vi "Stream Reader.vi"(7 "Popup? (F)":bool, 8 "error in (no error)":errorcluster, 10 "Signals in":refnum<class "ISignal.lvclass">[](array[class])) -> (0 "error out":errorcluster)   [LabVIEW 2022 SP3, in "StreamReader.lvlib"]
uses:
  <instrlib>/openDAQ/Examples/StreamReader/StreamReader.lvlib
  <instrlib>/openDAQ/Public/TypeDef/DomainMetadata.ctl
  <instrlib>/openDAQ/Public/Classes/ISignal/ISignal.lvclass
  C:/Program Files (x86)/National Instruments/LabVIEW 2022/instr.lib/openDAQ/Public/Classes/IComponent/IComponent.lvclass
  C:/Program Files (x86)/National Instruments/LabVIEW 2022/instr.lib/openDAQ/Public/Classes/IBaseObject/IBaseObject.lvclass
  <instrlib>/openDAQ/Examples/StreamReader/TypeDef/State.ctl
  <instrlib>/openDAQ/Public/Classes/IInstance/IInstance.lvclass
  C:/Program Files (x86)/National Instruments/LabVIEW 2022/instr.lib/openDAQ/Public/Classes/IDevice/IDevice.lvclass
  <instrlib>/openDAQ/Public/Classes/IDevice/IDevice.lvclass
  <instrlib>/openDAQ/Public/Classes/IStreamReader/IStreamReader.lvclass
  C:/Program Files (x86)/National Instruments/LabVIEW 2022/instr.lib/openDAQ/Public/Classes/IReader/IReader.lvclass
  <instrlib>/openDAQ/Public/Classes/IBaseObject/Polymorphic/queryInterface/queryDataDescriptorInterface.vi
  <instrlib>/openDAQ/Public/Classes/daqCoreTypes/IDict/IDict.lvclass
  <instrlib>/openDAQ/Public/Classes/IBaseObject/IBaseObject.lvclass
  <instrlib>/openDAQ/Public/Classes/IDataDescriptor/IDataDescriptor.lvclass
  <instrlib>/openDAQ/Public/Classes/IEventPacket/IEventPacket.lvclass
  <instrlib>/openDAQ/Public/Classes/daqUtils/daqUtils.lvlib
  <instrlib>/openDAQ/openDAQ.lvlib
  <instrlib>/openDAQ/Public/Classes/IReaderStatus/IReaderStatus.lvclass
  <instrlib>/openDAQ/Public/Classes/IComponent/IComponent.lvclass
  <instrlib>/openDAQ/Public/Classes/IReader/IReader.lvclass
panel:
  in  "Btn:StopMeasurement":bool
  in  "Online Buffer":i32=1000
  in  "Btn:StartMeasurement":bool
  in  "Btn:Stop":bool
  out "Iteration":i32
  out "DomainMetadata":T1
  in  "Global ID's":i32(listbox)
  out "XY Graph":T2(graph)
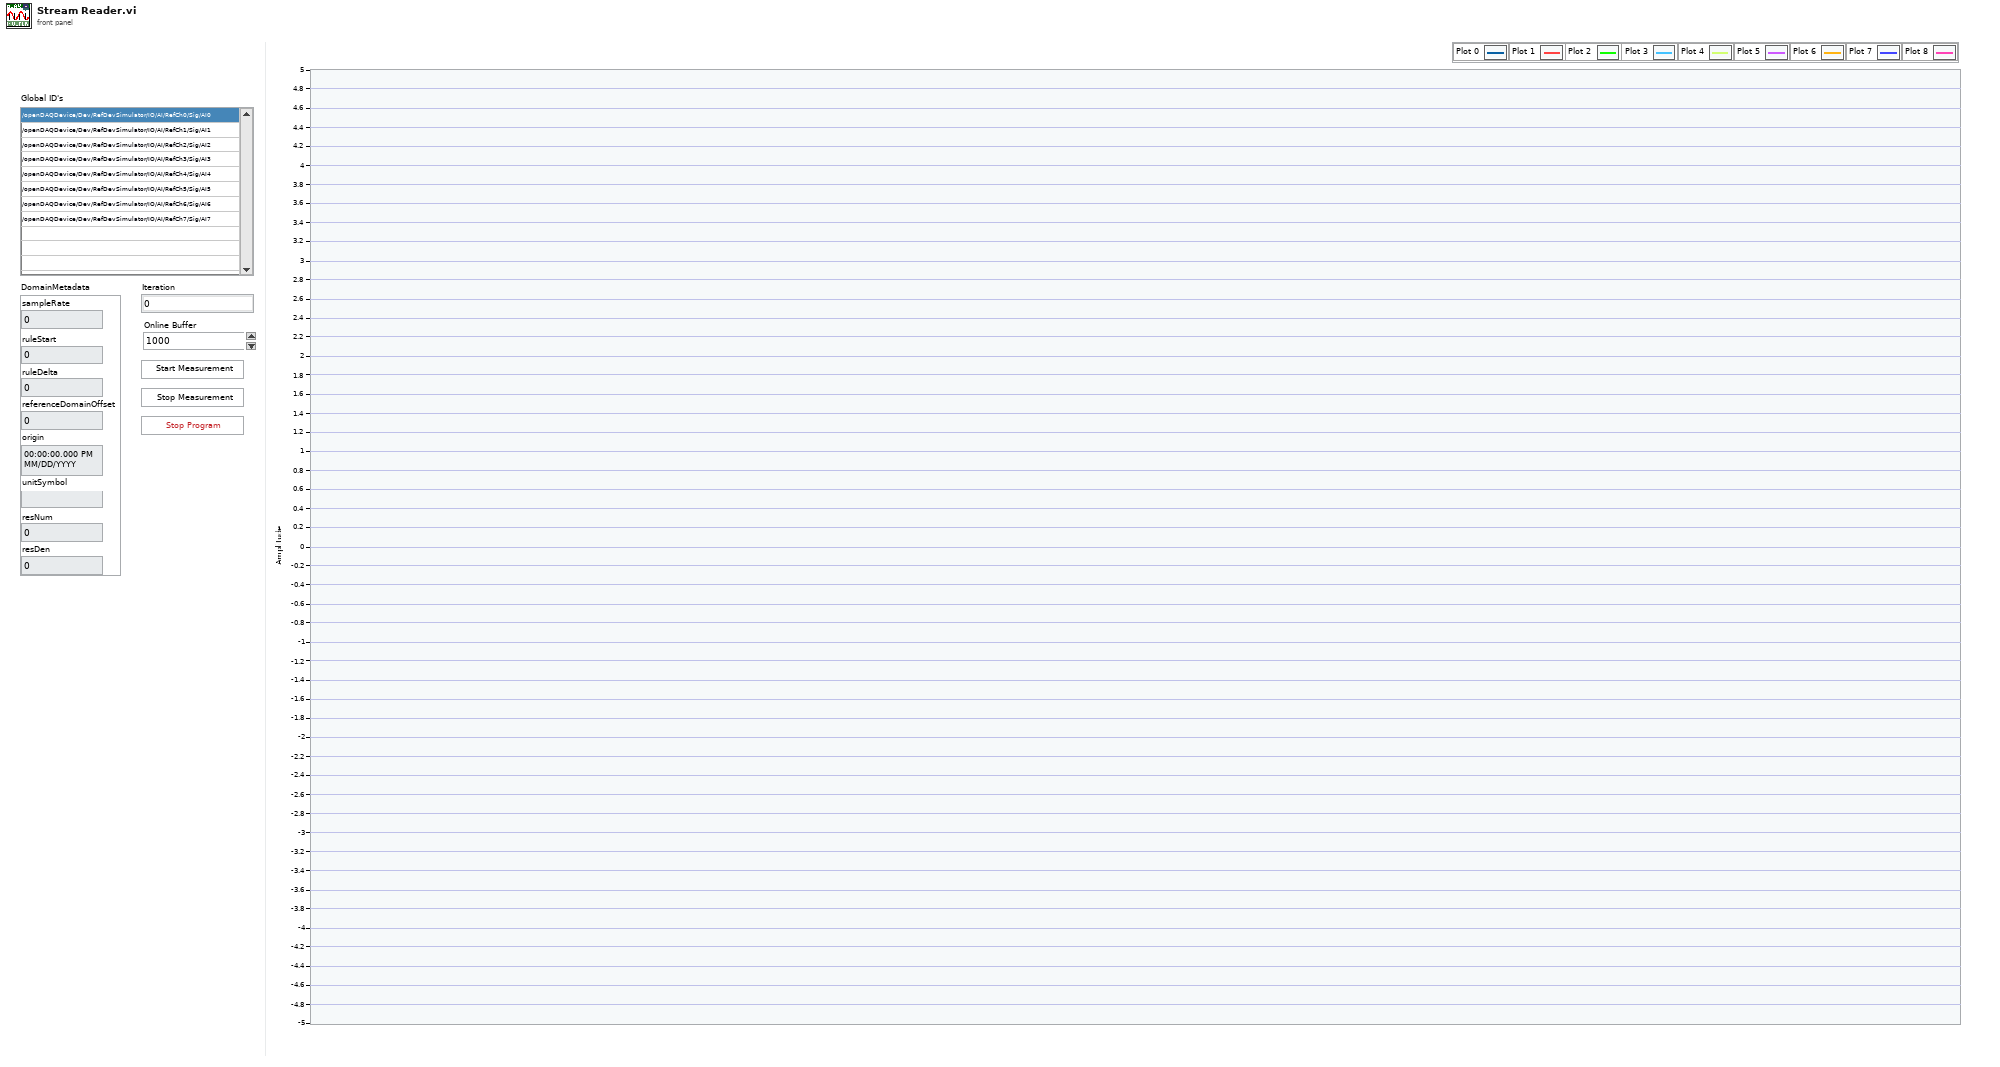
[diagram p1: front panel]
types:
  T1 = typedef "openDAQ.lvlib/DomainMetadata.ctl" = cluster{"sampleRate":i64, "ruleStart":i64, "ruleDelta":i64, "referenceDomainOffset":i64, "origin":timestamp, "unitSymbol":string, "resNum":i64, "resDen":i64}
  T2 = cluster{"Waveform Graph":timestamp[], "Waveform Graph":dbl[]}
  T3 = cluster{"Simulator":refnum<class "IInstance.lvclass">, "Instance":refnum<class "IInstance.lvclass">, "ConnectedDevice":refnum<class "IDevice.lvclass">, "Signals":refnum<class "ISignal.lvclass">[], "ChannelCount":i32, "StreamReader":refnum<class "IStreamReader.lvclass">}
  T4 = typedef "StreamReader.lvlib/State.ctl" = enum16{"INIT", "- SIMULATOR.setup", "IDLE", "- DAQ.start", "- DAQ.read", "- DAQ.end", "STOP", "ERROR"}
  T5 = enum16{"init", "read", "set sampleRate", "set ruleStart", "set ruleDelta", "set referenceDomainOffset", "set origin", "set unitSymbol", "set resNum", "set resDen", " calculate sampleRate"}
  T6 = enum8{"Enabled", "Disabled", "Disabled and Grayed Out"}
  T7 = cluster{"Value Buffer":dbl[], "Domain Buffer":i64[]}
  T8 = typedef "openDAQ.lvlib/ReadStatus.ctl" = u16
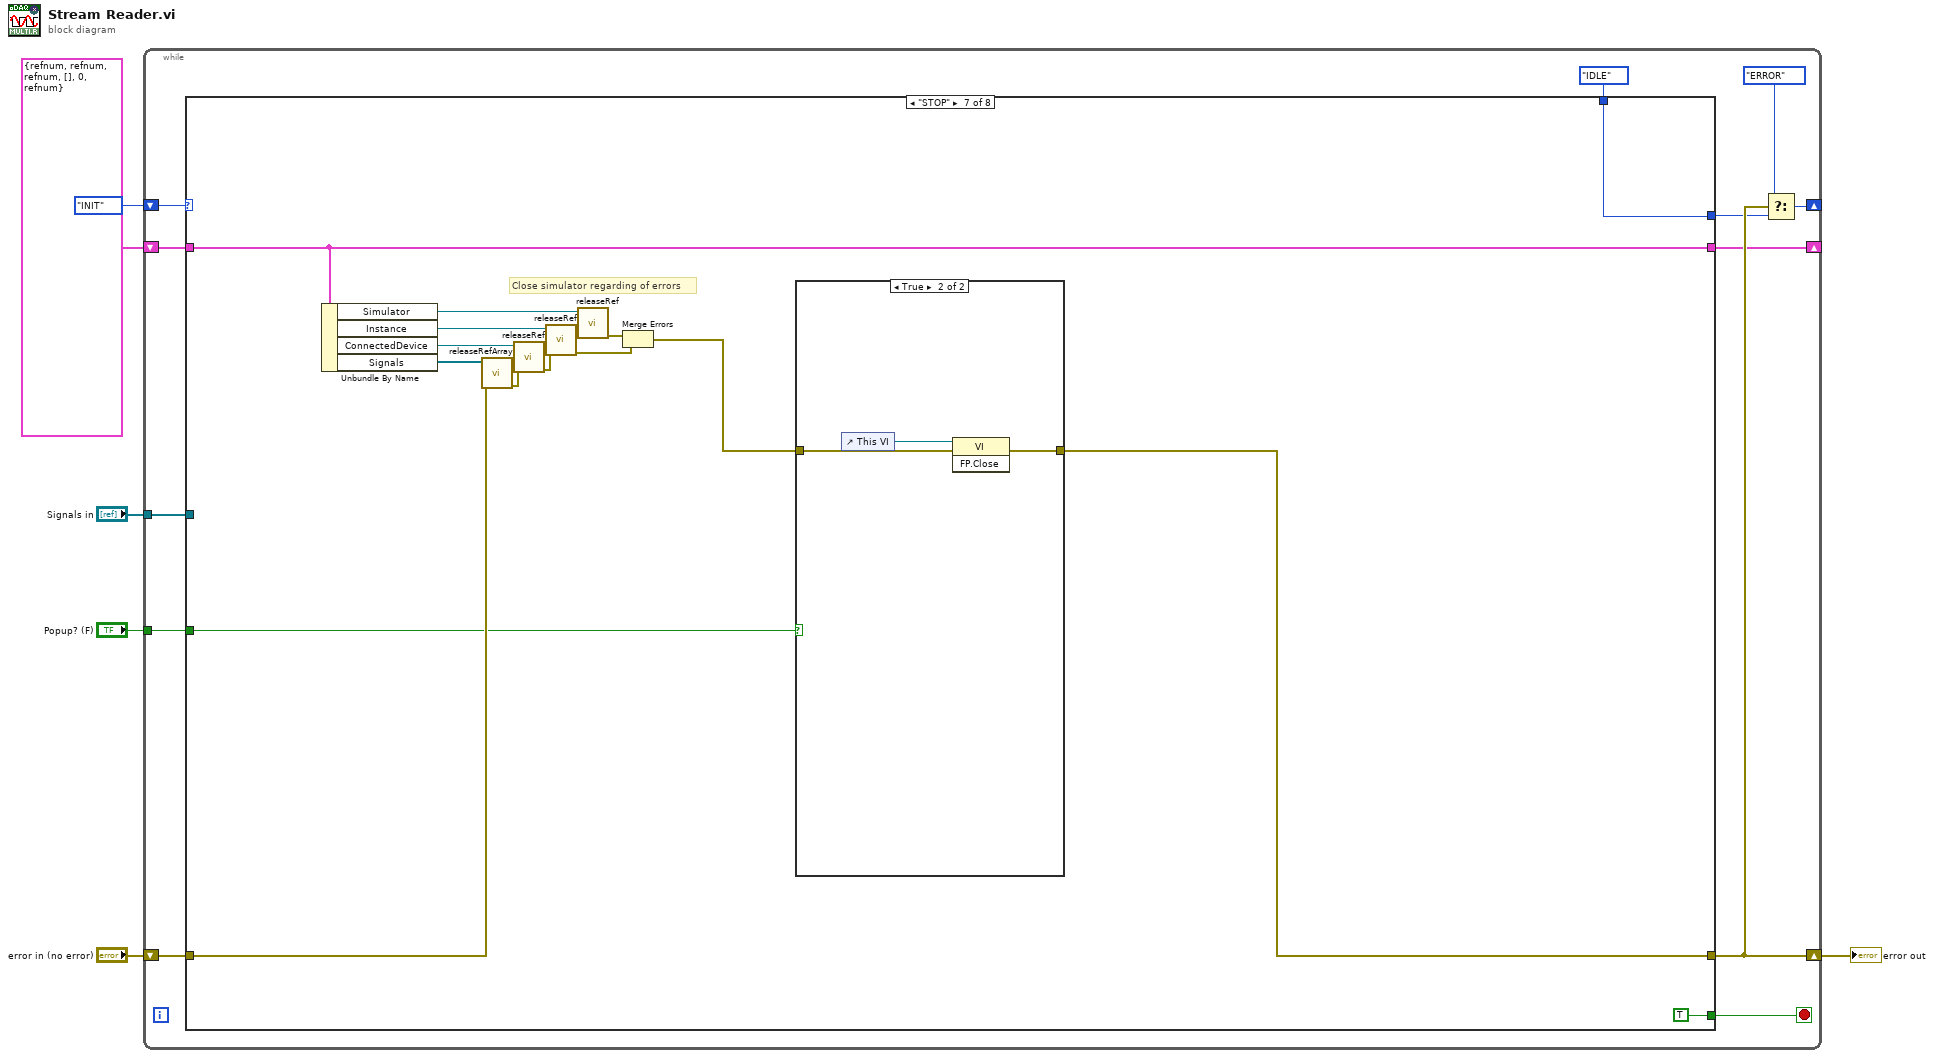
[diagram p0: block diagram]
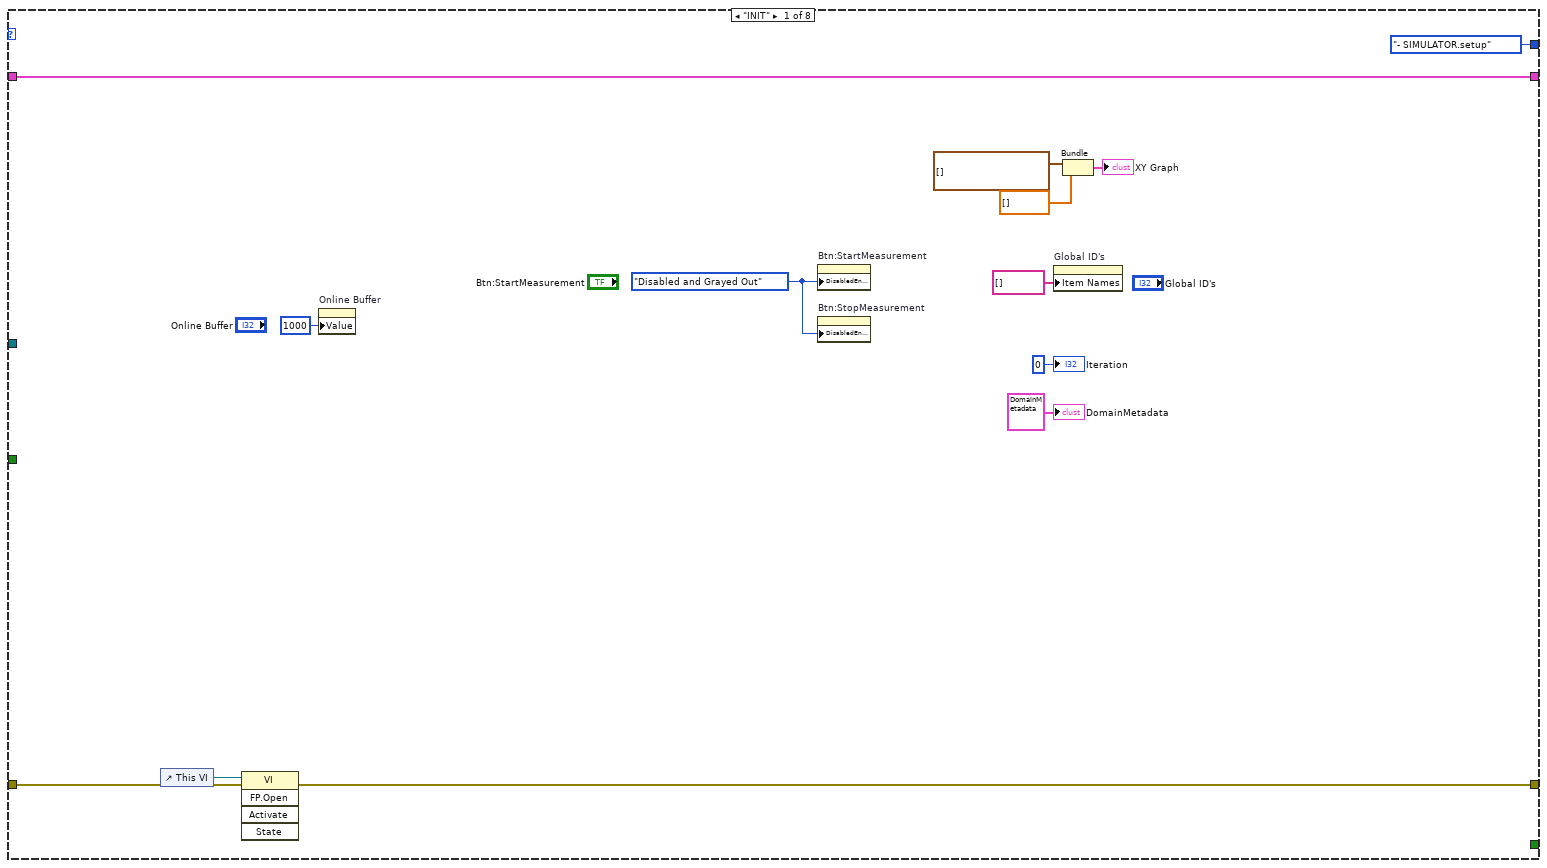
[diagram p2: hidden frame]
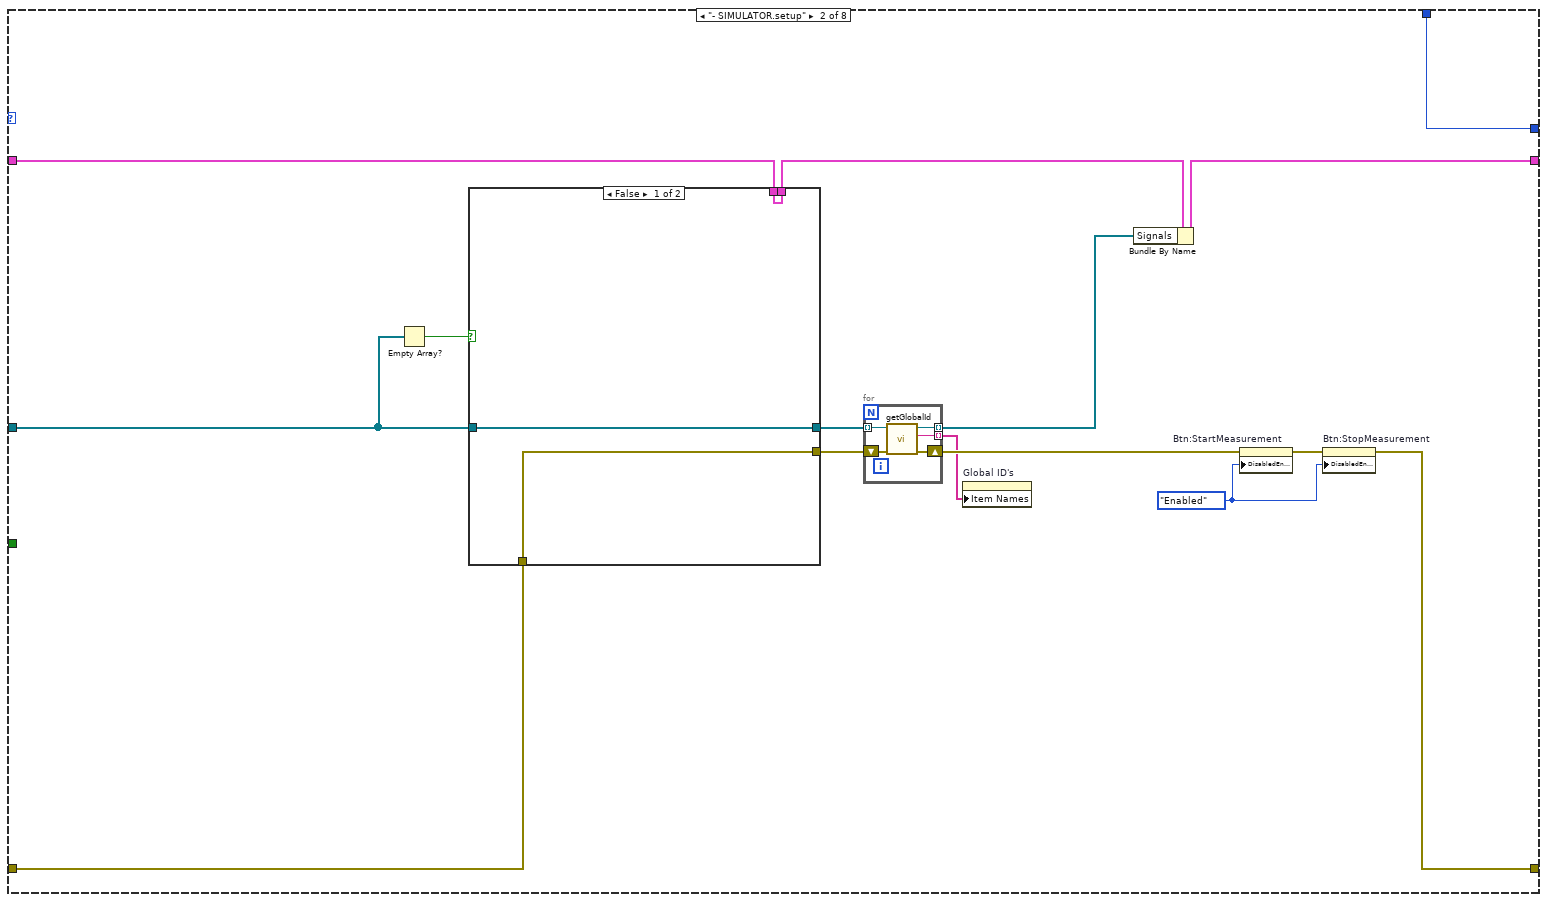
[diagram p3: hidden frame]
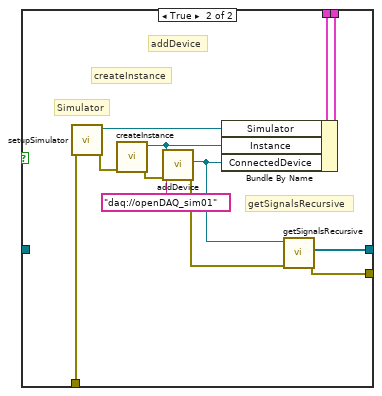
[diagram p4: hidden frame]
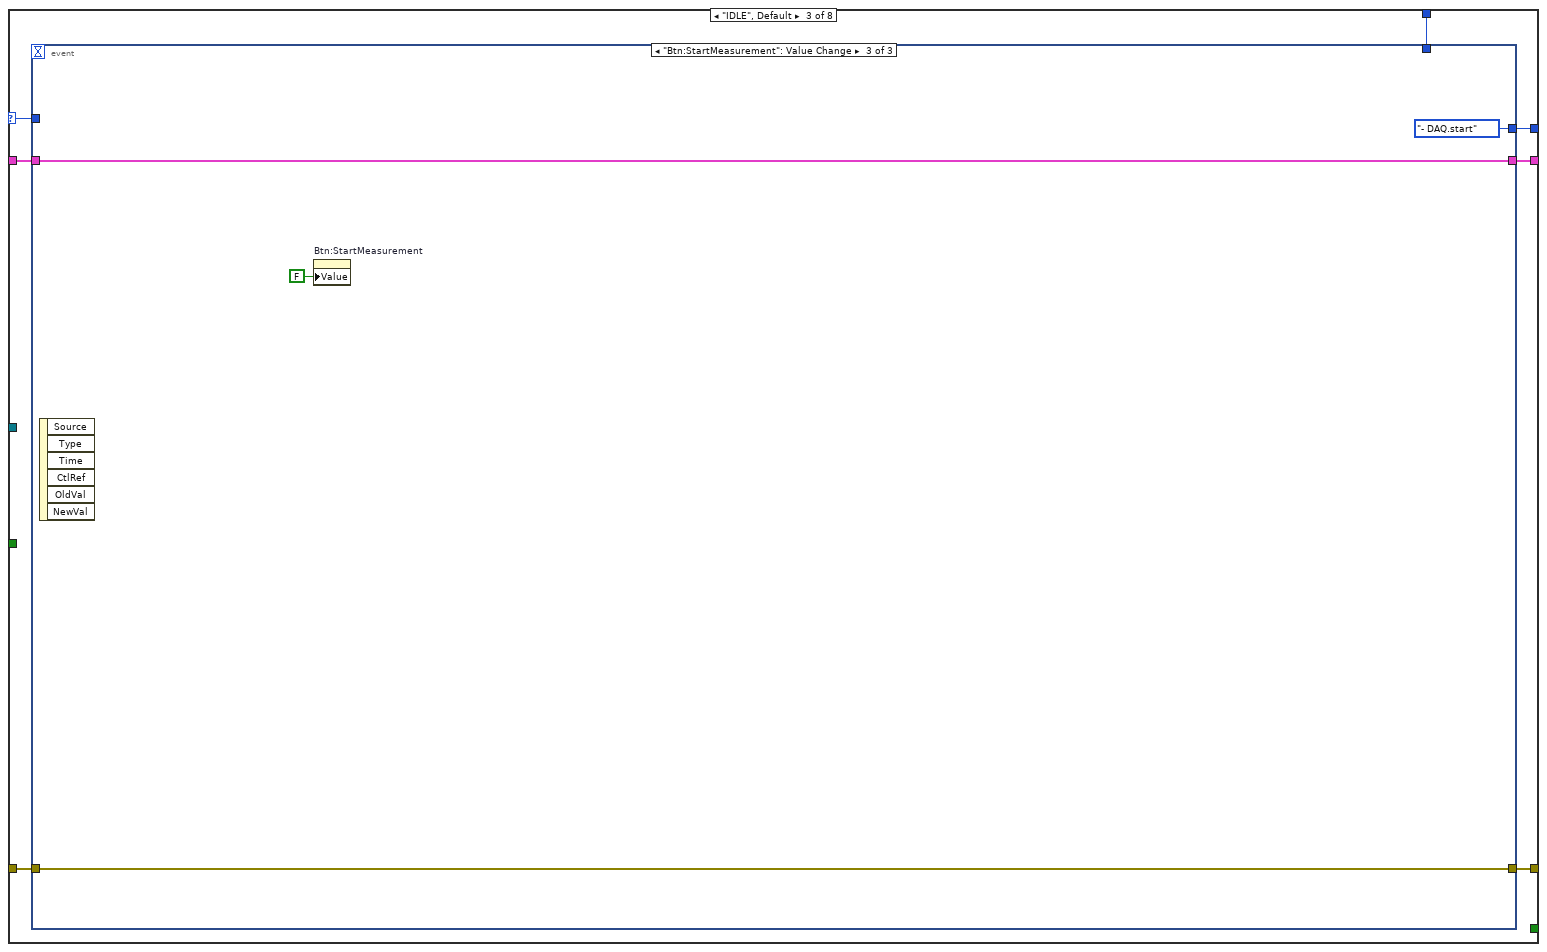
[diagram p5: hidden frame]
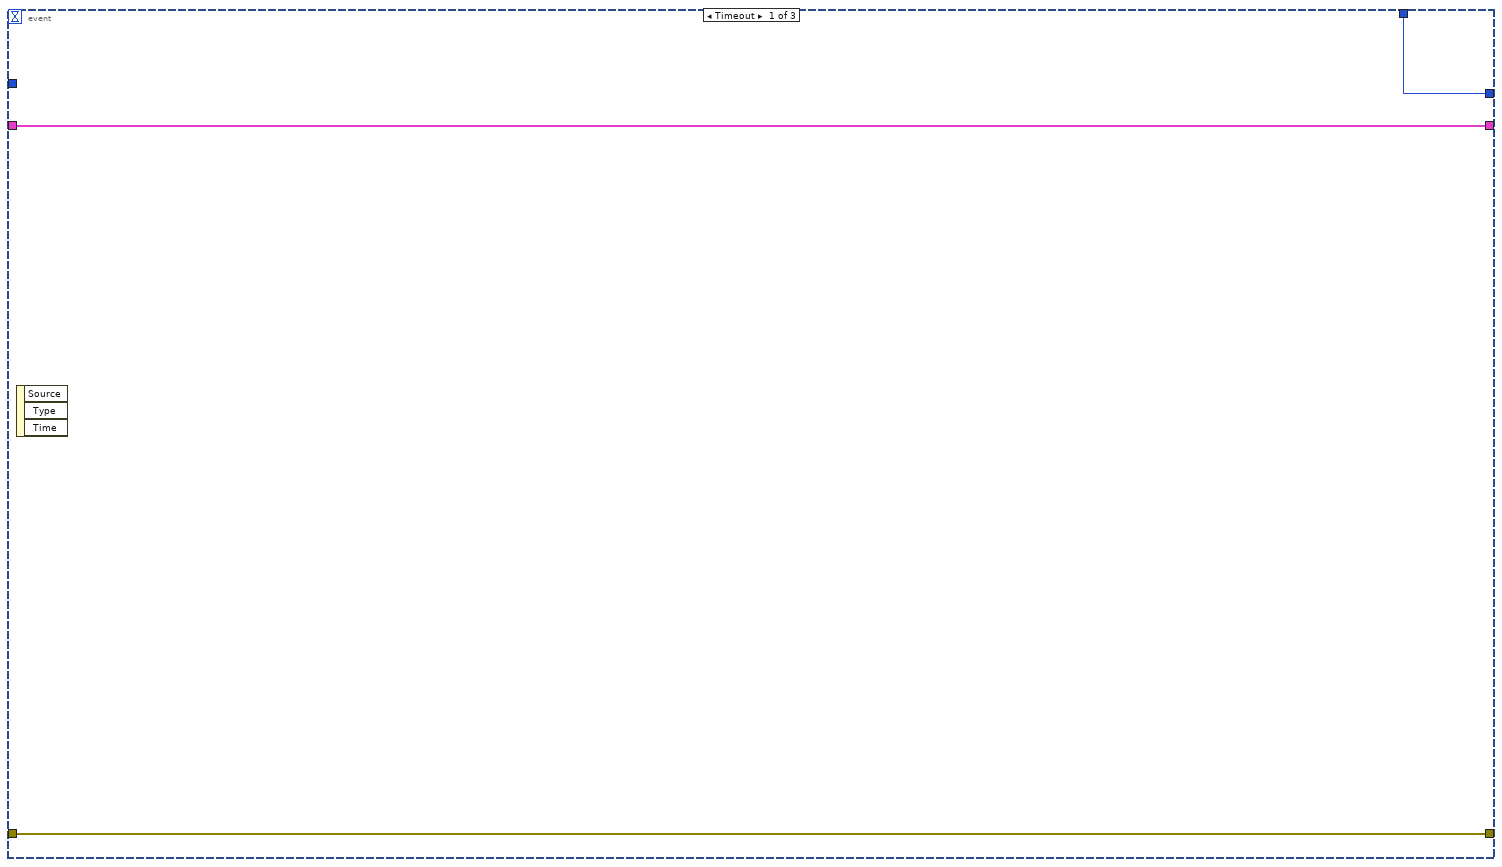
[diagram p6: hidden frame]
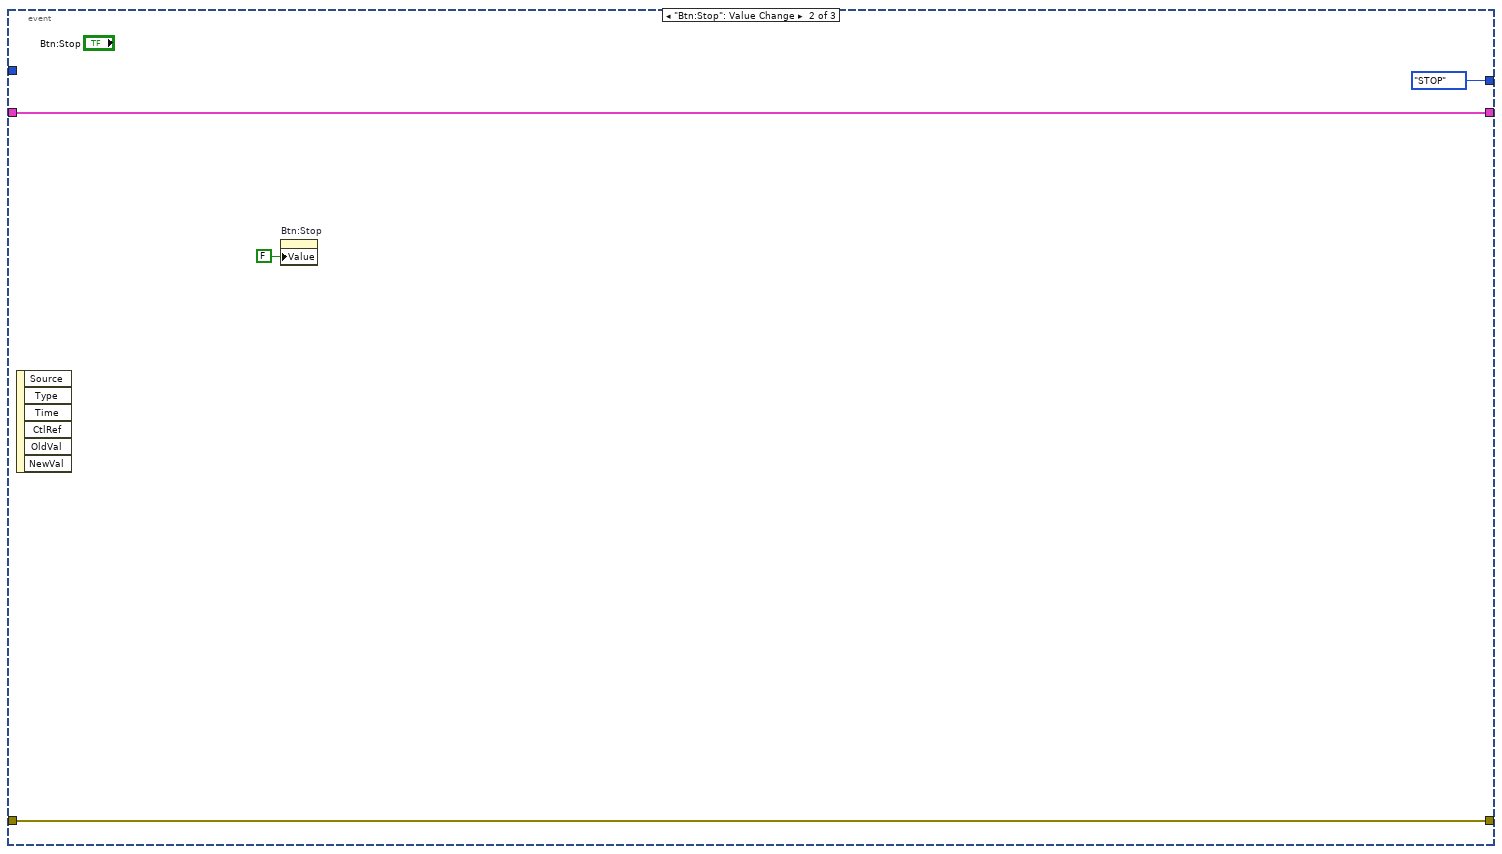
[diagram p7: hidden frame]
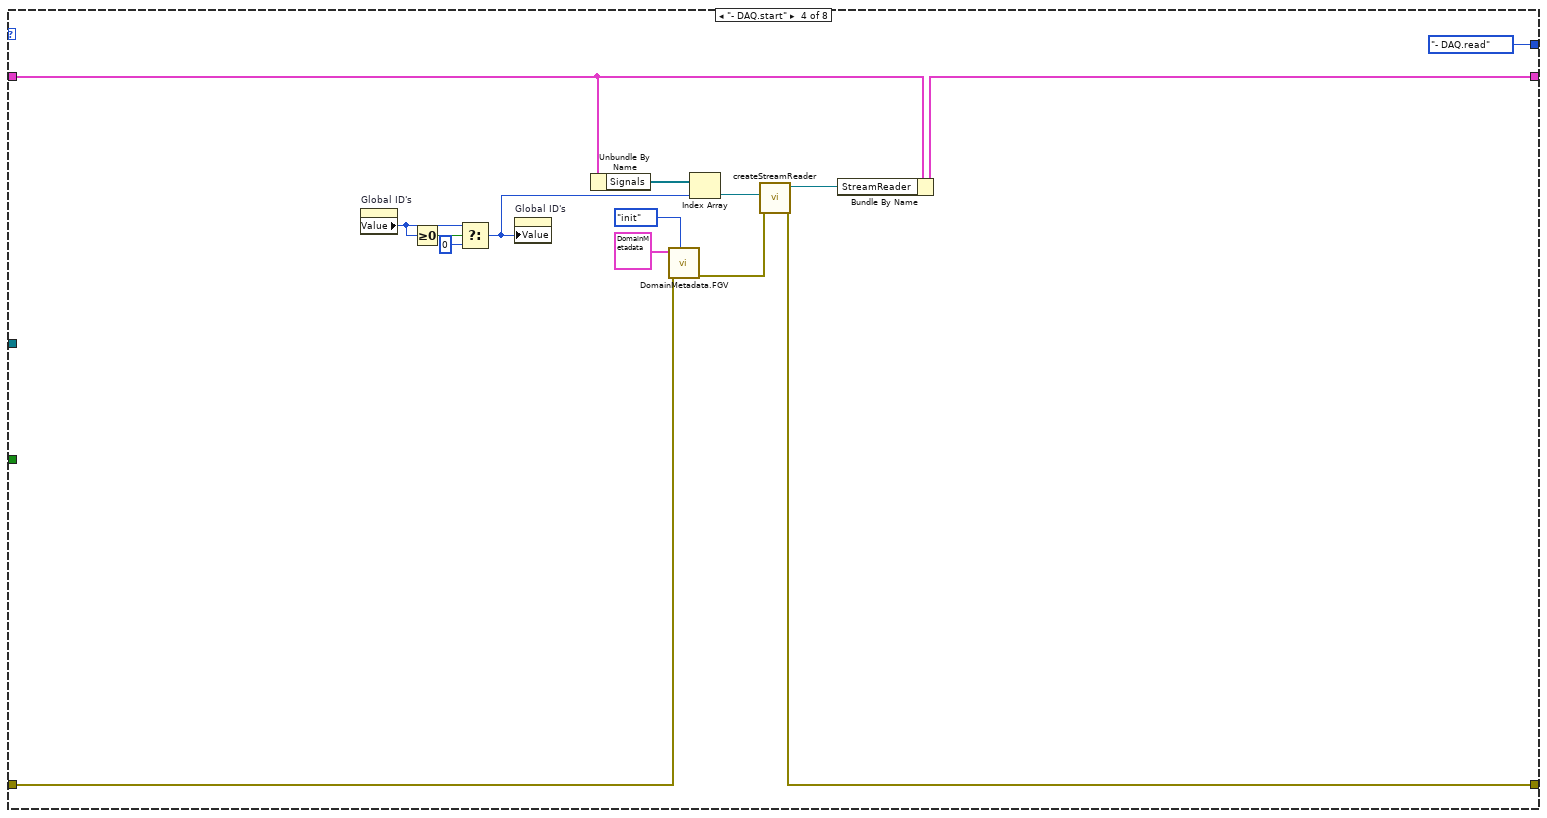
[diagram p8: hidden frame]
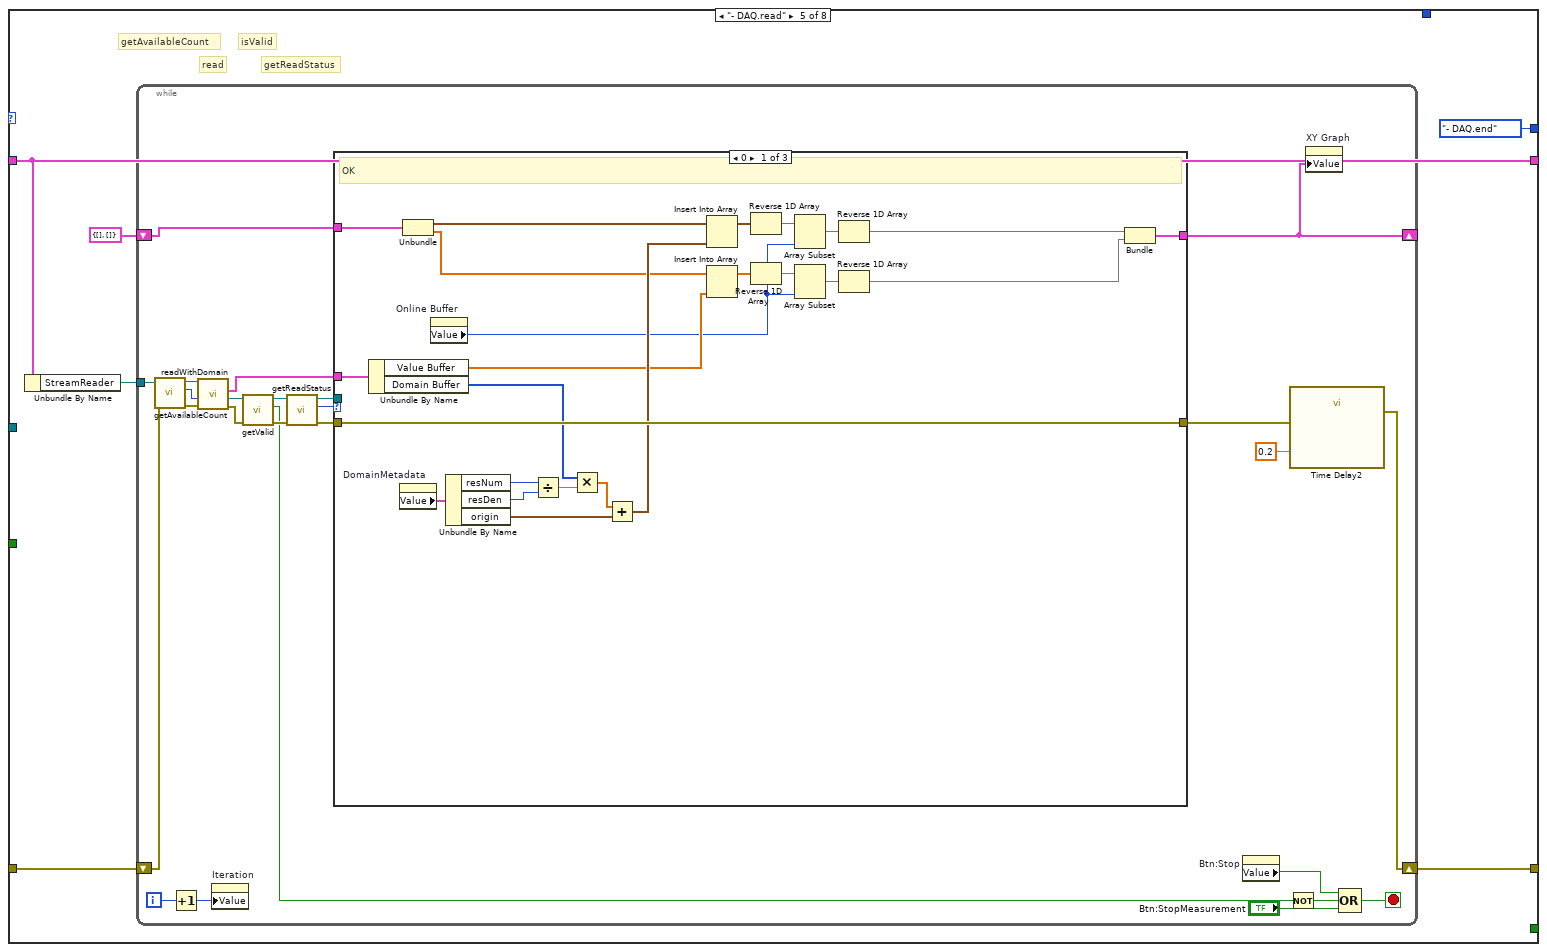
[diagram p9: hidden frame]
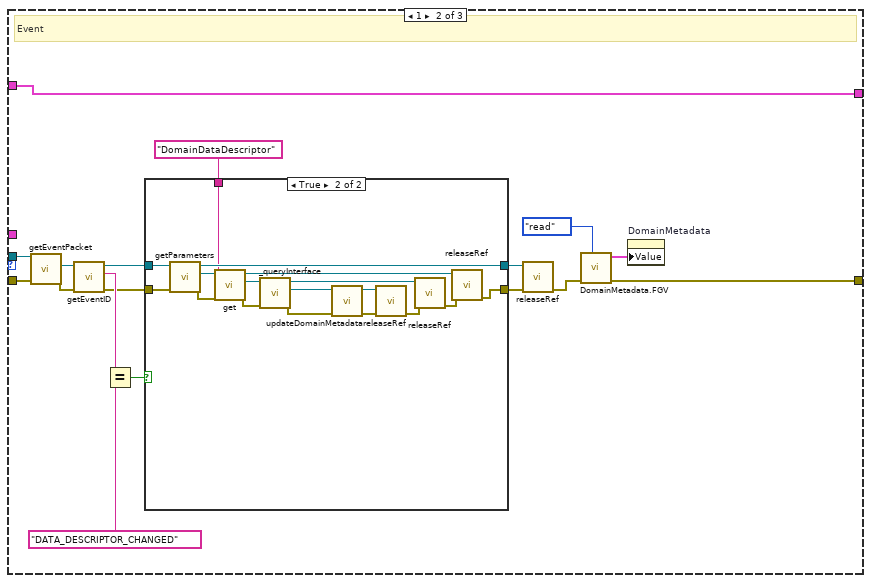
[diagram p10: hidden frame]
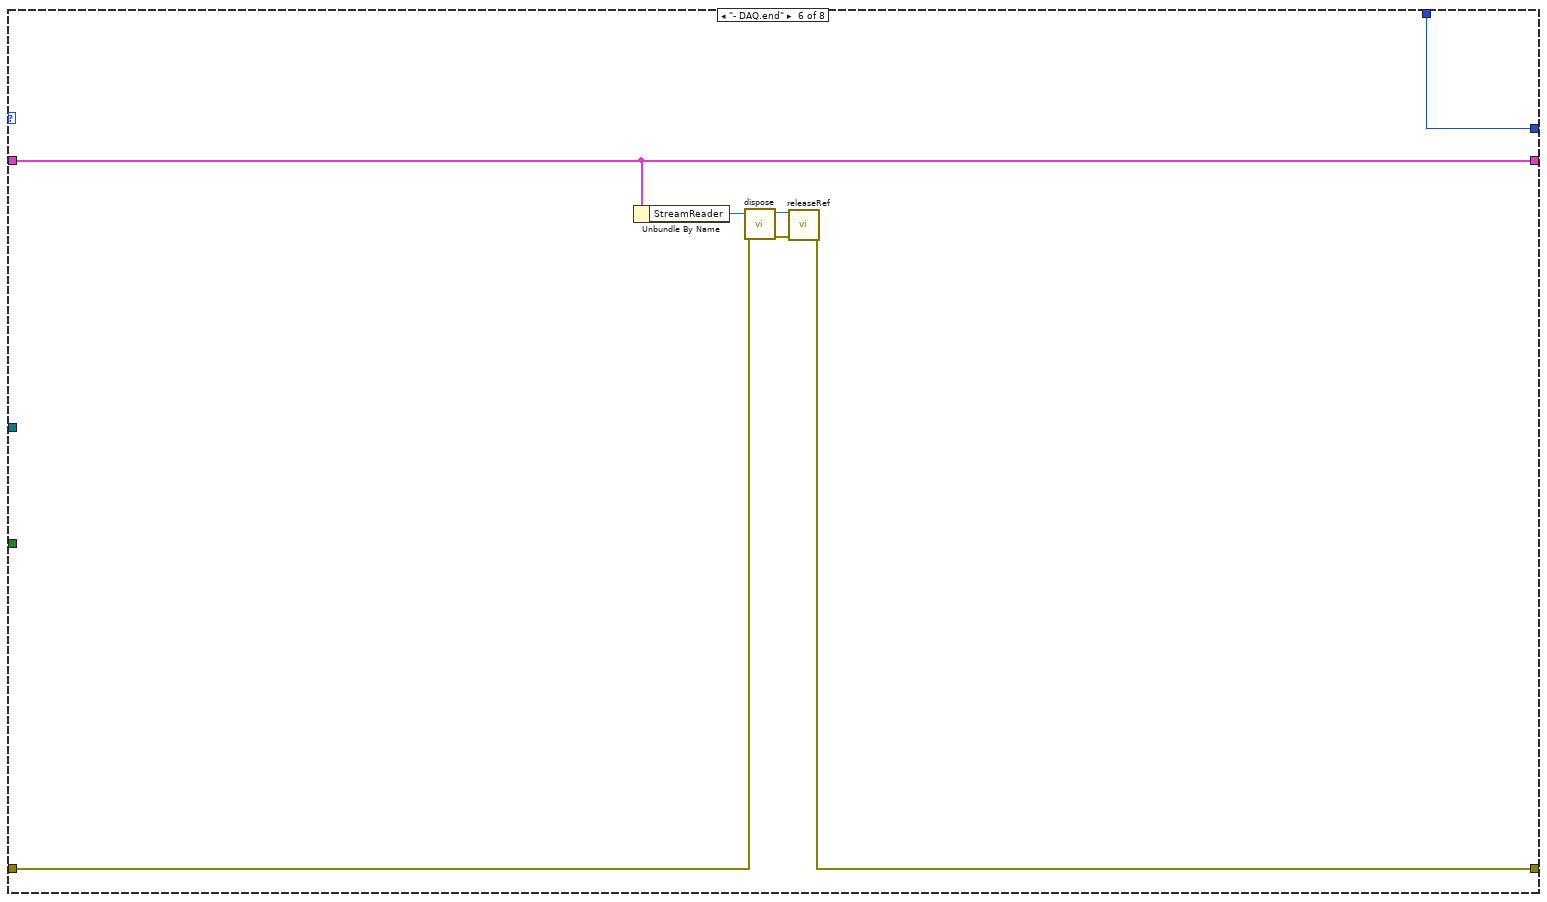
[diagram p13: hidden frame]
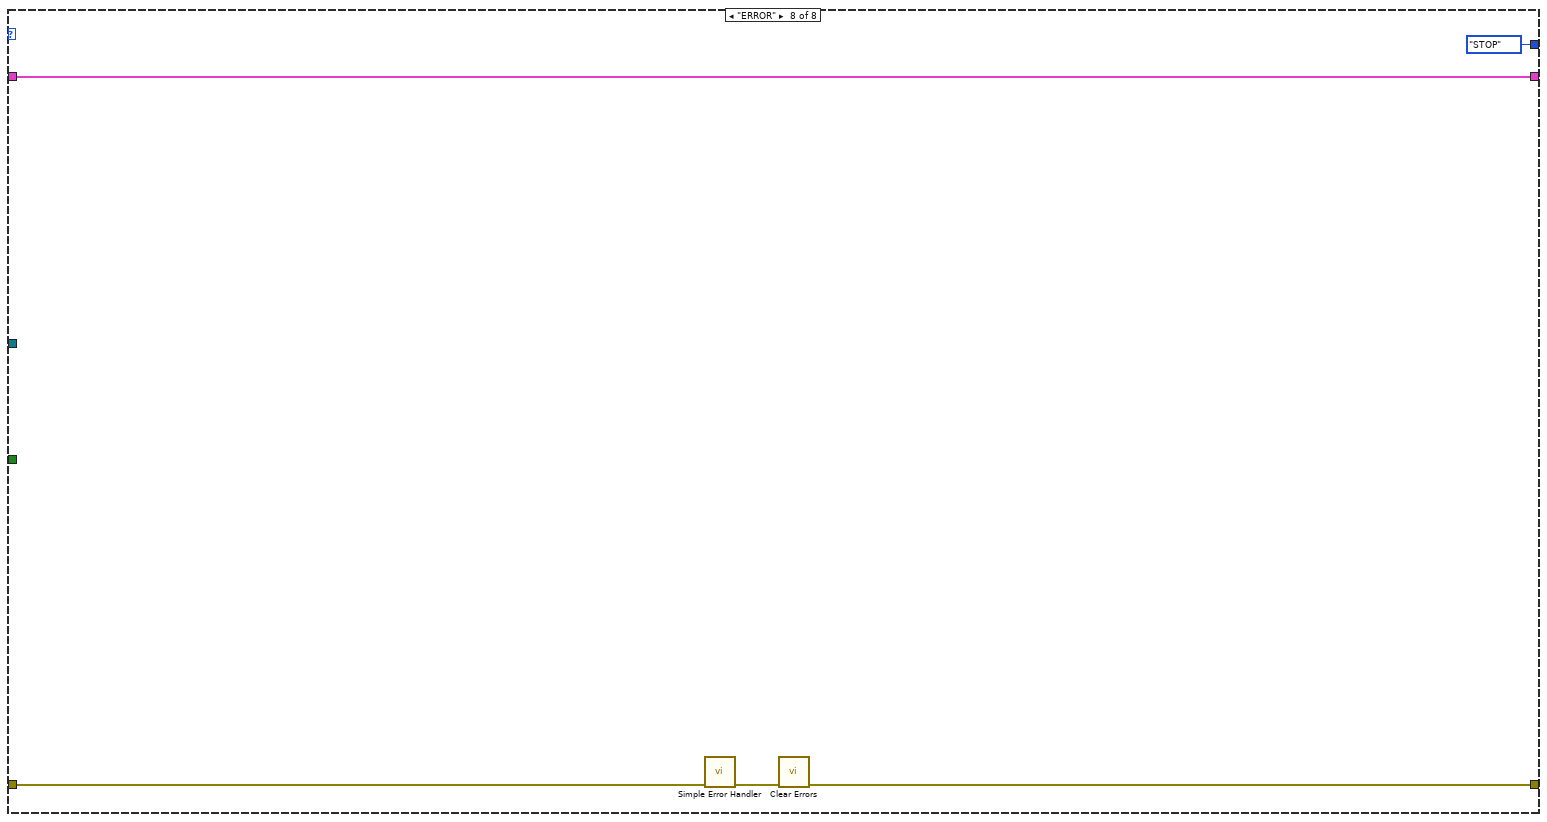
[diagram p15: hidden frame]
diagram:
  n1 = while {
    shift-right: [w11] -> _
    shift-left: State."INIT" -> [w17]
    shift-right: [w18] -> w2
    shift-left: "error in (no error)" -> [w14]
    shift-right: [w12] -> _
    shift-left: T3 {"Simulator"=refnum, "Instance"=refnum, "ConnectedDevice"=refnum, "Signals"=[], "ChannelCount"=0, "StreamReader"=refnum} -> [w13]
    tunnel: "Signals in" -> [w8]
    tunnel: "Popup? (F)" -> [w7]
    stop <- w16 stop-if-true
    n2 = case shown="\"STOP\"" w17 {
      selector: w17 -> [_ _ w73 _ _ _ _ _]
      tunnel: [State."- SIMULATOR.setup" w44 w71 State."- DAQ.read" State."- DAQ.end" w199 w203 State."STOP"] -> w10
      tunnel: [_ _ _ _ _ _ TRUE _] -> w16
      tunnel: State."IDLE" -> [_ w44 w72 _ _ w199 w203 _]
      tunnel: w14 -> [w24 w45 w70 w86 w103 w195 w205 w221]
      tunnel: [w23 w39 w69 w98 w102 w197 w200 w220] -> w18
      tunnel: w13 -> [w31 w43 w68 w95 w104 w198 w213 w223]
      tunnel: [w31 w41 w67 w93 w104 w198 w213 w223] -> w12
      tunnel: w8 -> [_ w36 _ _ _ _ _ _]
      tunnel: w7 -> [_ _ _ _ _ _ w202 _]
      frame "INIT" {
        w26 = T6."Disabled and Grayed Out" ("Disabled")
        n3 = control-ref of="This VI"() -> (w25:refnum<vi>)
        n4 = invoke class="VI" method="FP.Open"(reference=w25, error in=w24) -> (error out=w23:errorcluster)  [unwired: 3 in, 4 out]
        n5 = property on="Online Buffer" class="DigNum (strict)"("Value"=1000 ("Online Buffer")) -> ()  [unwired: 2 in, 2 out]
        n6 = property on="Btn:StartMeasurement" class="Bool (strict)"("DisabledEnum"=w26) -> ()  [unwired: 2 in, 2 out]
        n7 = property on="Btn:StopMeasurement" class="Bool"("DisabledEnum"=w26) -> ()  [unwired: 2 in, 2 out]
        n8 = property on="Global ID's" class="LstBox (strict)"("Item Names"=string[] [] ("Global ID's")) -> ()  [unwired: 2 in, 2 out]
        n9 = Bundle("Waveform Graph"=timestamp[] [], "Waveform Graph"=dbl[] []) -> (→"XY Graph":T2)  [unwired: 1 in]
        "Iteration" <- 0 ("Iteration")
        "DomainMetadata" <- T1 {"sampleRate"=0, "ruleStart"=0, "ruleDelta"=0, "referenceDomainOffset"=0, "origin"=timestamp(0 s since 1904-01-01), "unitSymbol"="", "resNum"=0, "resDen"=0} ("DomainMetadata")
      }
      frame "- SIMULATOR.setup" {
        w38 = T6."Enabled" ("Disabled")
        n10 = Empty Array?(array=w36) -> (empty?=w37:bool)
        n11 = case shown="False" w37 {
          tunnel: w45 -> [w53 w66]
          tunnel: w43 -> [w54 w60]
          tunnel: [w52 w56] -> w34
          tunnel: [w54 w57] -> w42
          tunnel: [w53 w55] -> w33
          tunnel: w36 -> [w52 _]
          frame False {
          }
          frame True {
            # "Simulator"
            # "addDevice"
            # "createInstance"
            # "getSignalsRecursive"
            n12 = call <instrlib>:"setupSimulator.vi"("error in (no error)"=w66) -> ("error out"=w63:errorcluster, "IInstance out"=w62:refnum<class "IInstance.lvclass">)  [unwired: 9 in]
            n13 = call <instrlib>:"createInstance.vi"("error in (no error)"=w63) -> ("error out"=w65:errorcluster, "IInstance out"=w61:refnum<class "IInstance.lvclass">)  [unwired: 9 in]
            n14 = call <instrlib>:"addDevice.vi"("error in (no error)"=w65, "ConnectionString in"="daq://openDAQ_sim01" ("modulePath"), "IDevice in"=w61) -> ("error out"=w59:errorcluster, "ConnectedDevice out"=w58:refnum<class "IDevice.lvclass">)  [unwired: 6 in, 1 out]
            n15 = Bundle By Name(cluster=w60, "Simulator"=w62, "Instance"=w61, "ConnectedDevice"=w58) -> (w57:T3)
            n16 = call <instrlib>:"getSignalsRecursive.vi"("error in (no error)"=w59, "IDevice in"=w58) -> ("error out"=w55:errorcluster, "Available Sigals out"=w56:refnum<class "ISignal.lvclass">[])  [unwired: 7 in, 1 out]
          }
        }
        n17 = for {
          tunnel: w34 -> [w51] mode=indexing
          tunnel: [w50] -> w32 mode=indexing
          tunnel: [w47] -> w35 mode=indexing
          shift-right: [w48] -> w46
          shift-left: w33 -> [w49]
          n18 = call <instrlib>:"getGlobalId.vi"("error in (no error)"=w49, "IComponent in"=w51) -> ("error out"=w48:errorcluster, "GlobalId out"=w47:string, "IComponent out"=w50:refnum<class "ISignal.lvclass">)  [unwired: 7 in]
        }
        n19 = property on="Global ID's" class="LstBox (strict)"("Item Names"=w35) -> ()  [unwired: 2 in, 2 out]
        n20 = Bundle By Name(cluster=w42, "Signals"=w32) -> (w41:T3)
        n21 = property on="Btn:StartMeasurement" class="Bool (strict)"(error in=w46, "DisabledEnum"=w38) -> (error out=w40:errorcluster)  [unwired: 1 in, 1 out]
        n22 = property on="Btn:StopMeasurement" class="Bool"(error in=w40, "DisabledEnum"=w38) -> (error out=w39:errorcluster)  [unwired: 1 in, 1 out]
      }
      frame "IDLE", Default {
        n23 = event shown="[2] \"Btn:StartMeasurement\": Value Change" {
          selector: _ -> [_ _ _]
          dyn-events: _ -> [_ _ _]
          timeout: _ -> [_ _ _]
          tunnel: w73 -> [_ _ _]
          tunnel: [w76 State."STOP" State."- DAQ.start"] -> w71
          tunnel: w72 -> [w76 _ _]
          tunnel: w70 -> [w75 w80 w82]
          tunnel: [w75 w80 w82] -> w69
          tunnel: w68 -> [w74 w79 w83]
          tunnel: [w74 w79 w83] -> w67
          event Timeout {
            n24 = event-data() -> ()  [unwired: 1 in, 3 out]
          }
          event "Btn:Stop": Value Change {
            n25 = event-data() -> ()  [unwired: 1 in, 6 out]
            n26 = property on="Btn:Stop" class="Bool (strict)"("Value"=FALSE ("Btn:Stop")) -> ()  [unwired: 2 in, 2 out]
          }
          event "Btn:StartMeasurement": Value Change {
            n27 = event-data() -> ()  [unwired: 1 in, 6 out]
            n28 = property on="Btn:StartMeasurement" class="Bool (strict)"("Value"=FALSE ("Btn:StartMeasurement")) -> ()  [unwired: 2 in, 2 out]
          }
        }
      }
      frame "- DAQ.start" {
        n29 = property on="Global ID's" class="LstBox (strict)"() -> ("Value"=w91:i32)  [unwired: 2 in, 2 out]
        n30 = Greater Or Equal To 0?(x=w91) -> (x >= 0?=w92:bool)
        n31 = Select(t=w91, s=w92, f=0) -> (s? t:f=w89:i32)
        n32 = property on="Global ID's" class="LstBox (strict)"("Value"=w89) -> ()  [unwired: 2 in, 2 out]
        n33 = Unbundle By Name(w95) -> ("Signals"=w97:refnum<class "ISignal.lvclass">[])
        n34 = call <instrlib>:"DomainMetadata.FGV.vi"("Case Select"=T5."init", "error in"=w86, "DomainMetadata in"=T1 {"sampleRate"=1, "ruleStart"=0, "ruleDelta"=1, "referenceDomainOffset"=0, "origin"=timestamp(0 s since 1904-01-01), "unitSymbol"="", "resNum"=0, "resDen"=0}) -> ("error out"=w85:errorcluster)  [unwired: 7 in, 1 out]
        n35 = Index Array(array=w97, index=w89) -> (element=w96:refnum<class "ISignal.lvclass">)
        n36 = call <instrlib>:"createStreamReader.vi"("error in (no error)"=w85, "connectedSignal"=w96) -> ("error out"=w98:errorcluster, "IStreamReader out"=w94:refnum<class "IStreamReader.lvclass">)  [unwired: 8 in]
        n37 = Bundle By Name(cluster=w95, "StreamReader"=w94) -> (w93:T3)
      }
      frame "- DAQ.read" {
        # "getReadStatus"
        # "isValid"
        # "read"
        # "getAvailableCount"
        n38 = Unbundle By Name(w104) -> ("StreamReader"=w101:refnum<class "IStreamReader.lvclass">)
        n39 = while {
          shift-right: [w127] -> w102
          shift-left: w103 -> [w115]
          tunnel: w101 -> [w118]
          shift-right: [w106] -> _
          shift-left: cluster{timestamp[], "Value Buffer":dbl[]} {[], "Value Buffer"=[]} -> [w109]
          i -> [w129]
          stop <- w123 stop-if-true
          n40 = call <instrlib>:"getAvailableCount.vi"("error in (no error)"=w115, "IReader in"=w118) -> ("error out"=w114:errorcluster, "Available Count"=w116:i32, "IReader out"=w117:refnum<class "IStreamReader.lvclass">)  [unwired: 7 in]
          n41 = Increment(x=w129) -> (x+1=w128:i32)
          n42 = call <instrlib>:"readWithDomain.vi"("error in (no error)"=w114, "bufferSize"=w116, "IStreamReader in"=w117) -> ("error out"=w121:errorcluster, "Reader Status out"=w120:refnum<class "IReaderStatus.lvclass">, "Read Buffers"=w108:T7)  [unwired: 5 in, 1 out]
          n43 = property on="Iteration" class="DigNum (strict)"("Value"=w128) -> ()  [unwired: 2 in, 2 out]
          n44 = call <instrlib>:"getValid.vi"("error in (no error)"=w121, "ReaderStatus in"=w120) -> ("error out"=w130:errorcluster, "isValid?"=w119:bool, "ReaderStatus out"=w113:refnum<class "IReaderStatus.lvclass">)  [unwired: 7 in]
          n45 = call <instrlib>:"getReadStatus.vi"("error in (no error)"=w130, "IReaderStatus in"=w113) -> ("error out"=w111:errorcluster, "ReadStatus"=w112:T8, "IReaderStatus out"=w110:refnum<class "IReaderStatus.lvclass">)  [unwired: 7 in]
          n46 = case shown="0" w112 {
            tunnel: w111 -> [w153 w170 w192]
            tunnel: w110 -> [_ w171 _]
            tunnel: w109 -> [w145 w167 w191]
            tunnel: w108 -> [w154 _ _]
            tunnel: [w133 w167 w191] -> w106
            tunnel: [w153 w157 w192] -> w107
            frame 0 {
              # "OK"
              n47 = Unbundle By Name(w154) -> ("Value Buffer"=w135:dbl[], "Domain Buffer"=w152:i64[])
              n48 = property on="DomainMetadata" class="Clust (strict)"() -> ("Value"=w148:T1)  [unwired: 2 in, 2 out]
              n49 = Unbundle(w145) -> (w142:timestamp[], "Value Buffer"=w136:dbl[])
              n50 = property on="Online Buffer" class="DigNum (strict)"() -> ("Value"=w134:i32)  [unwired: 2 in, 2 out]
              n51 = Unbundle By Name(w148) -> ("resNum"=w150:i64, "resDen"=w151:i64, "origin"=w146:timestamp)
              n52 = Divide(x=w150, y=w151) -> (x/y=w149:dbl)
              n53 = Multiply(x=w152, y=w149) -> (x*y=w147:dbl[])
              n54 = Add(x=w147, y=w146) -> (x+y=w141:timestamp[])
              n55 = Insert Into Array(array=w142, new element=w141) -> (w137:timestamp[])  [unwired: 1 in]
              n56 = Insert Into Array(array=w136, new element=w135) -> (w140:dbl[])  [unwired: 1 in]
              n57 = Reverse 1D Array(array=w137) -> (reversed array=w144:timestamp[])
              n58 = Reverse 1D Array(array=w140) -> (reversed array=w138:dbl[])
              n59 = Array Subset(array=w144, length=w134) -> (w143:timestamp[])  [unwired: 1 in]
              n60 = Array Subset(array=w138, length=w134) -> (w139:dbl[])  [unwired: 1 in]
              n61 = Reverse 1D Array(array=w143) -> (reversed array=w132:timestamp[])
              n62 = Reverse 1D Array(array=w139) -> (reversed array=w131:dbl[])
              n63 = Bundle(w132, w131) -> (w133:cluster{timestamp[], dbl[]})  [unwired: 1 in]
            }
            frame 1 {
              # "Event"
              n64 = call <instrlib>:"getEventPacket.vi"("error in (no error)"=w170, "IMultiReaderStatus in"=w171) -> ("error out"=w169:errorcluster, "EventPacket out"=w168:refnum<class "IEventPacket.lvclass">)  [unwired: 7 in, 1 out]
              n65 = call <instrlib>:"getEventID.vi"("error in (no error)"=w169, "IEventPacket in"=w168) -> ("error out"=w163:errorcluster, "EventID out"=w165:string, "IEventPacket out"=w160:refnum<class "IEventPacket.lvclass">)  [unwired: 7 in]
              n66 = Equal?(x=w165, y="DATA_DESCRIPTOR_CHANGED" ("x")) -> (x = y?=w164:bool)
              n67 = case shown="True" w164 {
                tunnel: w163 -> [w172 w178]
                tunnel: [w173 w177] -> w162
                tunnel: "DomainDataDescriptor" -> [_ w176]
                tunnel: w160 -> [w173 w175]
                tunnel: [w172 w174] -> w159
                frame False {
                }
                frame True {
                  n68 = call <instrlib>:"getParameters.vi"("error in (no error)"=w178, "IEventPacket in"=w175) -> ("error out"=w187:errorcluster, "Parameters out"=w190:refnum<class "IDict.lvclass">, "IEventPacket out"=w177:refnum<class "IEventPacket.lvclass">)  [unwired: 7 in]
                  n69 = call <instrlib>:"get.vi"("error in (no error)"=w187, "Key in"=w176, "IDict in"=w190) -> ("error out"=w188:errorcluster, "Value out"=w189:refnum<class "IBaseObject.lvclass">, "IDict out"=w182:refnum<class "IDict.lvclass">)  [unwired: 6 in]
                  n70 = call-poly <instrlib>:"_queryInterface.vi"("error in (no error)"=w188, "IBaseObject in"=w189) -> ("error out"=w186:errorcluster, "DataDescriptor out"=w185:refnum<class "IDataDescriptor.lvclass">, "IBaseObject out"=w181:refnum<class "IBaseObject.lvclass">)  [unwired: 7 in]
                  n71 = call <instrlib>:"updateDomainMetadata.vi"("error in"=w186, "IDataDescriptor in"=w185) -> ("error out"=w183:errorcluster, "IDataDescriptor out"=w184:refnum<class "IDataDescriptor.lvclass">)  [unwired: 8 in]
                  n72 = call-dynamic "releaseRef.vi"("error in (no error)"=w183, "IBaseObject in"=w184) -> ("error out"=w180:errorcluster)  [unwired: 9 in]
                  n73 = call-dynamic "releaseRef.vi"("error in (no error)"=w180, "IBaseObject in"=w181) -> ("error out"=w179:errorcluster)  [unwired: 9 in]
                  n74 = call-dynamic "releaseRef.vi"("error in (no error)"=w179, "IBaseObject in"=w182) -> ("error out"=w174:errorcluster)  [unwired: 9 in]
                }
              }
              n75 = call-dynamic "releaseRef.vi"("error in (no error)"=w159, "IBaseObject in"=w162) -> ("error out"=w158:errorcluster)  [unwired: 9 in]
              n76 = call <instrlib>:"DomainMetadata.FGV.vi"("Case Select"=T5."read", "error in"=w158) -> ("error out"=w157:errorcluster, "DomainMetadata out"=w155:T1)  [unwired: 8 in]
              n77 = property on="DomainMetadata" class="Clust (strict)"("Value"=w155) -> ()  [unwired: 2 in, 2 out]
            }
            frame Default {
              # "Failed, Unknown"
            }
          }
          n78 = property on="Btn:Stop" class="Bool (strict)"() -> ("Value"=w122:bool)  [unwired: 2 in, 2 out]
          n79 = Not(x=w119) -> (.not. x?=w125:bool)
          n80 = call "Time Delay2"("error in (no error)"=w107, "Delay Time (s)"=0.2) -> ("error out"=w127:errorcluster)  [unwired: 9 in]
          n81 = property on="XY Graph" class="XYGraph (strict)"("Value"=w106) -> ()  [unwired: 2 in, 2 out]
          n82 = Compound Arithmetic op=OR(w122, w125, "Btn:StopMeasurement") -> (w123:bool)
        }
      }
      frame "- DAQ.end" {
        n83 = Unbundle By Name(w198) -> ("StreamReader"=w194:refnum<class "IStreamReader.lvclass">)
        n84 = call-dynamic "dispose.vi"("error in (no error)"=w195, "IBaseObject in"=w194) -> ("error out"=w196:errorcluster, "IBaseObject out"=w193:refnum<class "IBaseObject.lvclass">)  [unwired: 8 in]
        n85 = call-dynamic "releaseRef.vi"("error in (no error)"=w196, "IBaseObject in"=w193) -> ("error out"=w197:errorcluster)  [unwired: 9 in]
      }
      frame "STOP" {
        # "Close simulator regarding of errors"
        n86 = Unbundle By Name(w213) -> ("Simulator"=w210:refnum<class "IInstance.lvclass">, "Instance"=w211:refnum<class "IInstance.lvclass">, "ConnectedDevice"=w212:refnum<class "IDevice.lvclass">, "Signals"=w206:refnum<class "ISignal.lvclass">[])
        n87 = call <instrlib>:"releaseRefArray.vi"("error in (no error)"=w205, "IBaseObject in"=w206) -> ("error out"=w204:errorcluster)  [unwired: 9 in]
        n88 = call-dynamic "releaseRef.vi"("error in (no error)"=w204, "IBaseObject in"=w212) -> ("error out"=w209:errorcluster)  [unwired: 9 in]
        n89 = call-dynamic "releaseRef.vi"("error in (no error)"=w209, "IBaseObject in"=w211) -> ("error out"=w207:errorcluster)  [unwired: 9 in]
        n90 = call-dynamic "releaseRef.vi"("IBaseObject in"=w210) -> ("error out"=w208:errorcluster)  [unwired: 10 in]
        n91 = Merge Errors(w208, w207) -> (w201:errorcluster)
        n92 = case shown="True" w202 {
          tunnel: w201 -> [w215 w217]
          tunnel: [w215 w216] -> w200
          frame False {
          }
          frame True {
            n93 = control-ref of="This VI"() -> (w218:refnum<vi>)
            n94 = invoke class="VI" method="FP.Close"(reference=w218, error in=w217) -> (error out=w216:errorcluster)  [unwired: 1 in, 2 out]
          }
        }
      }
      frame "ERROR" {
        n95 = call <vilib>:"Simple Error Handler.vi"("error in (no error)"=w221) -> ("error out"=w222:errorcluster)  [unwired: 4 in, 4 out]
        n96 = call <vilib>:"Clear Errors.vi"("error in (no error)"=w222) -> ("error out"=w220:errorcluster)  [unwired: 5 in, 1 out]
      }
    }
    n97 = Select(t=State."ERROR", s=w18, f=w10) -> (s? t:f=w11:T4)
  }
  "error out" <- w2
